vi "waveform demo.vi"() -> ()   [LabVIEW 2018]
uses:
  <instrlib>/Agilent 33XXX Series/Agilent 33XXX Series.lvlib
panel:
  out "Waveform Graph":waveform(dbl)(graph)
  out "Waveform Chart":waveform(dbl)(graph)
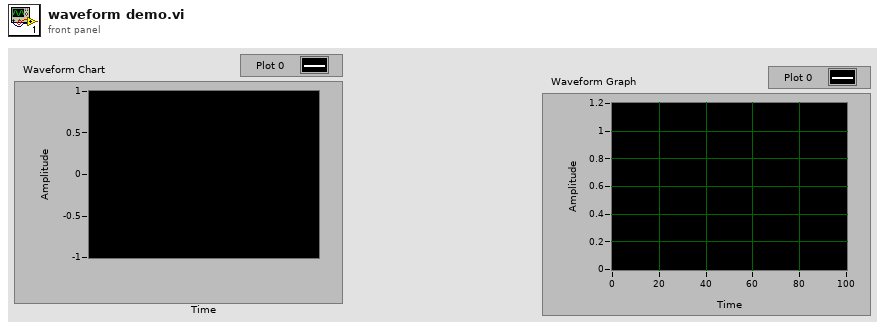
[diagram p1: front panel]
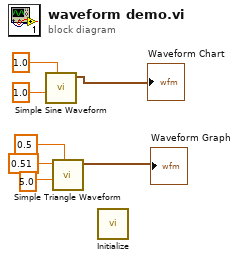
[diagram p0: block diagram]
diagram:
  n1 = call "Simple Sine Waveform.vi"("amplitude"=1.0, "n cycles"=1.0) -> ("sine waveform"=→"Waveform Chart":waveform(dbl))  [unwired: 9 in]
  n2 = call "Simple Triangle Waveform.vi"("amplitude"=0.5, "n cycles"=5.0, "offset"=0.51) -> ("triangle waveform"=→"Waveform Graph":waveform(dbl))  [unwired: 8 in]
  n3 = call <instrlib>:"Initialize.vi"() -> ()  [unwired: 10 in, 2 out]
